vi "DUPLICATE ITEM.vi"(11 "REFERENCES":T1) -> ()   [LabVIEW 2019]
uses:
  Controls/References Cluster.ctl
  <vilib>/userDefined/High Color/IMAQdx.ctl
  Controls/Custom Calendar/Custom Calendar.xctl
  Controls/Table Data Types/Inventory Data Type.ctl
  <vilib>/addons/database/Connection.llb/DB Tools Open Connec (String).vi
  <vilib>/addons/database/_DB Variant To Data/Database Variant To Data.xnode
  <vilib>/addons/database/NI_Database_API.lvlib
types:
  T1 = typedef "References Cluster.ctl" = cluster{"MAIN PAGES":refnum<vi>, "ADD/EDIT ITEM REFERENCES":cluster{"Identifier":refnum<vi>, "BYU ICN #":refnum<vi>, "Item Description":refnum<vi>, "Comments":refnum<vi>, "Checked Out Date":refnum<vi>, "Due Date":refnum<vi>, "Check Out Location":refnum<vi>, "Reminder Count":refnum<vi>, "Most Recent Reminder Date":refnum<vi>, "BYU ID #":refnum<vi>, "Building/Room":refnum<vi>, "Location in Room":refnum<vi>, "Manual":refnum<vi>, "Manufacturer":refnum<vi>, "Model #":refnum<vi>, "Serial #":refnum<vi>, "Date Acquired":refnum<vi>, "ADD/EDIT ITEM LABEL":refnum<vi>, "ARCHIVE ITEM":refnum<vi>, "Archive Item Inputs":refnum<vi>, "Reminder Notes":refnum<vi>, "DUPLICATE ITEM":refnum<vi>}, "ADD/EDIT USER REFERENCES":cluster{"BYU ID # (##-###-####)":refnum<vi>, "First Name":refnum<vi>, "Last Name":refnum<vi>, "Phone Number (###-###-####)":refnum<vi>, "Email":refnum<vi>, "Department":refnum<vi>, "Graduation Status":refnum<vi>, "Anticipated Graduation Year":refnum<vi>, "Credit Score":refnum<vi>, "Date Added":refnum<vi>, "Graduation Clearance Date":refnum<vi>, "Picture File Name":refnum<vi>, "ADD/EDIT USER LABEL":refnum<vi>, "Department Map":refnum<vi>, "Status Map":refnum<vi>, "Anticipated Graduation Year Map":refnum<vi>, "User Agreement":refnum<vi>, "User Comments":refnum<vi>, "Camera":refnum<vi>}, "RETURN ITEM REFERENCES":cluster{"Item or Person:":refnum<vi>, "Search Return Results":refnum<vi>, "What are you searching for?":refnum<vi>}, "SEARCH DATABASE REFERENCES":cluster{"What to Search For:":refnum<vi>, "Where to Search":refnum<vi>, "Column to Search In":refnum<vi>, "Column to Sort By":refnum<vi>, "Search Database Results":refnum<vi>, "Inventory Column Selector":refnum<vi>, "User Column Selector":refnum<vi>, "Inventory Archive Column Selector":refnum<vi>, "User Archive Column Selector":refnum<vi>, "Sales Tracking Column Selector":refnum<vi>, "Checked In Archive Column Selector":refnum<vi>, "Restore User":refnum<vi>, "Date Range":refnum<vi>, "Dates Less Than":refnum<vi>, "Dates Greater Than":refnum<vi>, "Search Print Receipt":refnum<vi>, "Edit Sale Description":refnum<vi>}, "USER ITEMS REFERENCES":cluster{"USER'S INFORMATION":refnum<vi>, "User's Checked Out Items":refnum<vi>, "User Info Comments":refnum<vi>, "SEE USER INFO COMMENTS":refnum<vi>}, "EDIT ITEMS REFERENCES":cluster{"New Check Out Location":refnum<vi>, "Items to Edit":refnum<vi>, "Edit Items Due Date":refnum<vi>, "New Reminder Notes":refnum<vi>, "New Item Description":refnum<vi>}, "CHECK OUT ITEMS REFERENCES":cluster{"Enter Item:":refnum<vi>, "Check Out Items Due Date":refnum<vi>, "Check Out Location":refnum<vi>, "Items to be Checked Out":refnum<vi>, "Possible Items":refnum<vi>, "Altered Item Description":refnum<vi>}, "TRANSFER ITEMS REFERENCES":cluster{"Search Parameter":refnum<vi>, "What to Match":refnum<vi>, "Matching Individuals":refnum<vi>, "Items to be Transferred":refnum<vi>}, "SETTINGS REFERENCES":cluster{"PSC Database Settings":refnum<vi>, "PSC Sales Item Spreadsheet":refnum<vi>}, "PSC SALES REFERENCES":cluster{"BYU ID CARD #":refnum<vi>, "Sale Description":refnum<vi>, "Scan or Enter Item Name":refnum<vi>, "Items to be Sold":refnum<vi>, "Grand Total":refnum<vi>, "Item List":refnum<vi>}}
  T2 = typedef "Inventory Data Type.ctl" = cluster{"Identifier":string, "BYU ICN #":string, "Item Description":string, "Comments":string, "Checked Out Date":string, "Due Date":string, "Check Out Location":string, "Reminder Count":i32, "Most Recent Reminder Date":string, "BYU ID #":string, "Building/Room":string, "Location in Room":string, "Manual":string, "Manufacturer":string, "Model #":string, "Serial #":string, "Date Acquired":string, "Reminder Notes":string}
  T3 = cluster{"Identifier":refnum<vi>, "BYU ICN #":refnum<vi>, "Item Description":refnum<vi>, "Comments":refnum<vi>, "Checked Out Date":refnum<vi>, "Due Date":refnum<vi>, "Check Out Location":refnum<vi>, "Reminder Count":refnum<vi>, "Most Recent Reminder Date":refnum<vi>, "BYU ID #":refnum<vi>, "Building/Room":refnum<vi>, "Location in Room":refnum<vi>, "Manual":refnum<vi>, "Manufacturer":refnum<vi>, "Model #":refnum<vi>, "Serial #":refnum<vi>, "Date Acquired":refnum<vi>, "ADD/EDIT ITEM LABEL":refnum<vi>, "ARCHIVE ITEM":refnum<vi>, "Archive Item Inputs":refnum<vi>, "Reminder Notes":refnum<vi>, "DUPLICATE ITEM":refnum<vi>}
  T4 = typedef "NI_Database_API.lvlib/Conn ObjectReference.ctl" = refnum<k1>
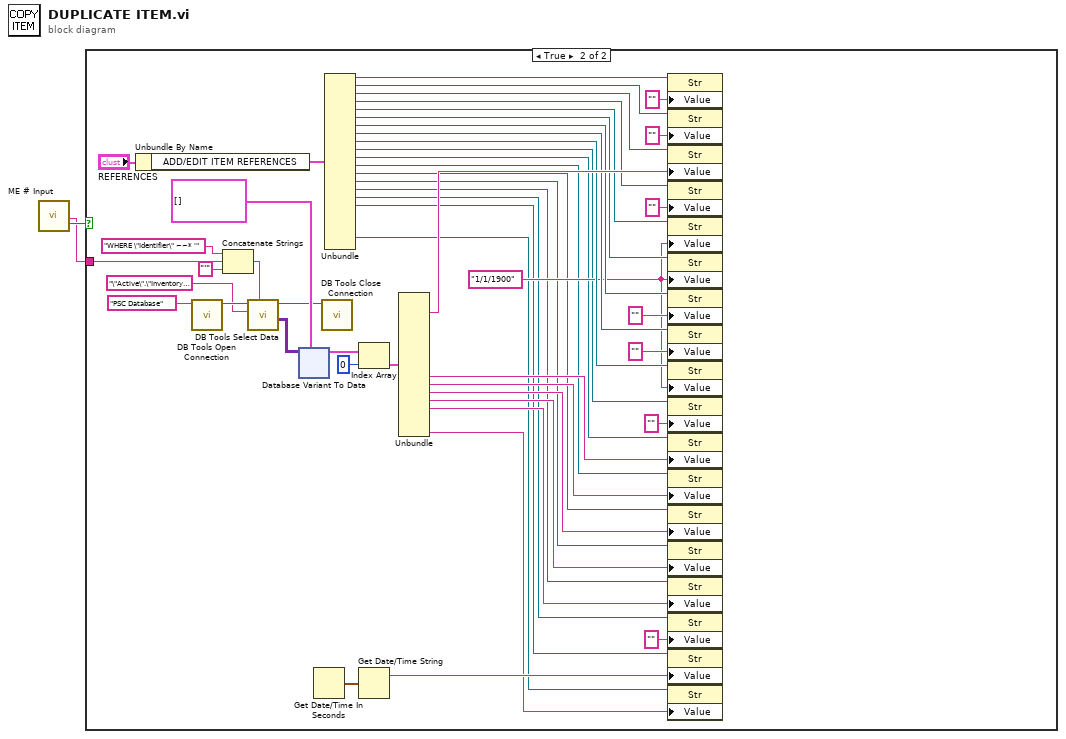
[diagram p0: block diagram]
diagram:
  n1 = call "ME # Input"() -> ("ME # Input"=w1:string, "OK"=w2:bool)  [unwired: 17 in, 1 out]
  n2 = case shown="True" w2 {
    tunnel: w1 -> [_ w49]
    frame False {
    }
    frame True {
      w22 = "1/1/1900" ("Value")
      n3 = Unbundle By Name("REFERENCES") -> ("ADD/EDIT ITEM REFERENCES"=w39:T3)
      n4 = call-poly <vilib>:"DB Tools Open Connection.vi"("connection information"="PSC Database") -> ("connection reference"=w51:T4)  [unwired: 7 in, 1 out]
      n5 = Concatenate Strings("WHERE \"Identifier\" ~~* '", w49, "'" ("string")) -> (w46:string)
      n6 = call <vilib>:"DB Tools Select Data.vi"("condition"=w46, "table"="\"Active\".\"Inventory\"", "connection reference"=w51) -> ("data"=w45:variant[][], "connection reference out"=w40:T4)  [unwired: 3 in, 1 out]
      n7 = xnode "Database Variant To Data"("database variant"=w45, "type"=T2[] [] ("Array")) -> ("data"=w43:T2[])  [unwired: 1 in, 1 out]
      n8 = Get Date/Time In Seconds() -> (seconds since 1Jan1904=w6:timestamp)
      n9 = call <vilib>:"DB Tools Close Connection.vi"("connection reference"=w40) -> ()  [unwired: 6 in, 1 out]
      n10 = Unbundle(w39) -> ("Identifier"=w38:refnum<vi>, "BYU ICN #"=w35:refnum<vi>, "Item Description"=w33:refnum<vi>, "Comments"=w31:refnum<vi>, "Checked Out Date"=w29:refnum<vi>, "Due Date"=w28:refnum<vi>, "Check Out Location"=w27:refnum<vi>, "Reminder Count"=w25:refnum<vi>, "Most Recent Reminder Date"=w23:refnum<vi>, "BYU ID #"=w21:refnum<vi>, "Building/Room"=w19:refnum<vi>, "Location in Room"=w17:refnum<vi>, "Manual"=w15:refnum<vi>, "Manufacturer"=w13:refnum<vi>, "Model #"=w11:refnum<vi>, "Serial #"=w9:refnum<vi>, "Date Acquired"=w7:refnum<vi>, "Reminder Notes"=w4:refnum<vi>)  [unwired: 4 out]
      n11 = Index Array(array=w43, index=0) -> (element=w37:T2)
      n12 = Get Date/Time String(seconds (now)=w6) -> (date string=w5:string)  [unwired: 2 in, 1 out]
      n13 = Unbundle(w37) -> ("Item Description"=w32:string, "Building/Room"=w18:string, "Location in Room"=w16:string, "Manual"=w14:string, "Manufacturer"=w12:string, "Model #"=w10:string, "Reminder Notes"=w3:string)  [unwired: 11 out]
      n14 = property class="Str"(reference=w38, "Value"="") -> ()  [unwired: 1 in, 2 out]
      n15 = property class="Str"(reference=w35, "Value"="") -> ()  [unwired: 1 in, 2 out]
      n16 = property class="Str"(reference=w33, "Value"=w32) -> ()  [unwired: 1 in, 2 out]
      n17 = property class="Str"(reference=w31, "Value"="") -> ()  [unwired: 1 in, 2 out]
      n18 = property class="Str"(reference=w29, "Value"=w22) -> ()  [unwired: 1 in, 2 out]
      n19 = property class="Str"(reference=w28, "Value"=w22) -> ()  [unwired: 1 in, 2 out]
      n20 = property class="Str"(reference=w27, "Value"="") -> ()  [unwired: 1 in, 2 out]
      n21 = property class="Str"(reference=w25, "Value"="") -> ()  [unwired: 1 in, 2 out]
      n22 = property class="Str"(reference=w23, "Value"=w22) -> ()  [unwired: 1 in, 2 out]
      n23 = property class="Str"(reference=w21, "Value"="") -> ()  [unwired: 1 in, 2 out]
      n24 = property class="Str"(reference=w19, "Value"=w18) -> ()  [unwired: 1 in, 2 out]
      n25 = property class="Str"(reference=w17, "Value"=w16) -> ()  [unwired: 1 in, 2 out]
      n26 = property class="Str"(reference=w15, "Value"=w14) -> ()  [unwired: 1 in, 2 out]
      n27 = property class="Str"(reference=w13, "Value"=w12) -> ()  [unwired: 1 in, 2 out]
      n28 = property class="Str"(reference=w11, "Value"=w10) -> ()  [unwired: 1 in, 2 out]
      n29 = property class="Str"(reference=w9, "Value"="") -> ()  [unwired: 1 in, 2 out]
      n30 = property class="Str"(reference=w7, "Value"=w5) -> ()  [unwired: 1 in, 2 out]
      n31 = property class="Str"(reference=w4, "Value"=w3) -> ()  [unwired: 1 in, 2 out]
    }
  }
